vi "Mouse Up Event.vi"(4 "User Parameter":T1, 5 "Event Data":T3, 6 "PaneRef":refnum<vi>, 7 "Event Common Data":cluster{"Source":T4, "Type":T5, "Time":u32} {"Source" items=["LabVIEW UI"=0, "ActiveX"=1, "User Event"=25]}) -> ()   [LabVIEW 2020]
uses:
  <vilib>/event_ctls.llb/eventsource.ctl
  <vilib>/event_ctls.llb/lveventtype.ctl
  <vilib>/Utility/miscctls.llb/LVPoint32TypeDef.ctl
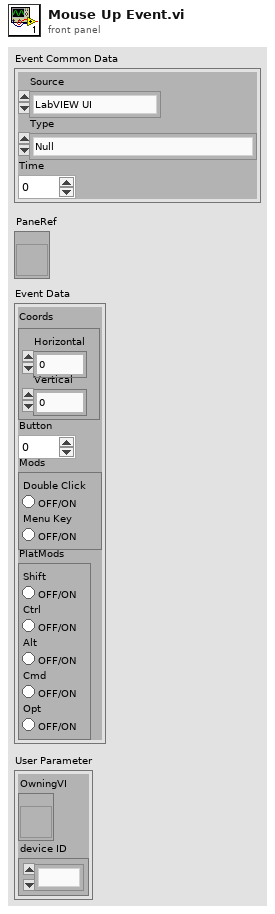
[diagram p1: front panel]
types:
  T1 = cluster{"OwningVI":refnum<vi>, "device ID":refnum<k1>}
  T2 = typedef "LVPoint32TypeDef.ctl" = cluster{"Horizontal":i32, "Vertical":i32}
  T3 = cluster{"Coords":T2, "Button":u16, "Mods":cluster{"Double Click":bool, "Menu Key":bool}, "PlatMods":cluster{"Shift":bool, "Ctrl":bool, "Alt":bool, "Cmd":bool, "Opt":bool}}
  T4 = typedef "eventsource.ctl" = u32
  T5 = typedef "lveventtype.ctl" = enum32{"Null", "Timeout", "Annotation Menu Selection", "Annotation Menu Selection?", "App Instance Close", "App Instance Close?", "Autoscale Range Change", "Bookmark Info Change", "Cell Edit", "Cell Edit?", "Cursor Grab", "Cursor Grab?", "Cursor Menu Selection", "Cursor Menu Selection?", "Cursor Move", "Cursor Release", "Data Change", "Direction Change", "Display State Change", "Drag Ended", "Drag Enter", "Drag Leave", "Drag Over", "Drag Source Update", "Drag Starting", "Drag Starting?", "Drop", "Exec State Change", "Key Down", "Key Down?", "Key Repeat", "Key Repeat?", "Key Up", "Listbox Double Click", "Menu Activation?", "Menu Selection (App)", "Menu Selection? (App)", "Menu Selection (User)", "Mouse Down", "Mouse Down?", "Mouse Enter", "Mouse Leave", "Mouse Move", "Mouse Up", "Mouse Wheel", "NI Security User Change (App)", "Pane Size", "Panel Close", "Panel Close?", "Panel Resize", "Plot Attribute Change", "Scale Range Change", "Shortcut Menu Activation?", "Shortcut Menu Selection (App)", "Shortcut Menu Selection? (App)", "Shortcut Menu Selection (User)", "Tree Double Click", "Tree Drag", "Tree Drag?", "Tree Drop", "Tree Drop?", "Tree Item Close", "Tree Item Close?", "Tree Item Open", "Tree Item Open?", "User Event", "Value Change"}
  T6 = typedef "LVRectTypeDef.ctl" = cluster{"Left":i16, "Top":i16, "Right":i16, "Bottom":i16}
  T7 = enum32{"Invalid", "Standard", "Closed", "Hidden", "Minimized", "Maximized"}
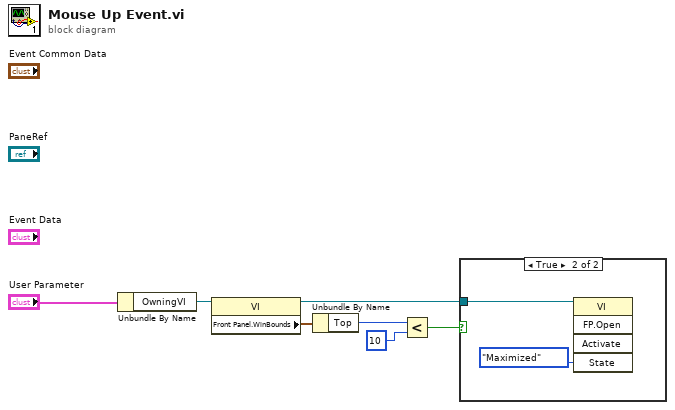
[diagram p0: block diagram]
diagram:
  n1 = Unbundle By Name("User Parameter") -> ("OwningVI"=w6:refnum<vi>)
  n2 = property class="VI"(reference=w6) -> (reference out=w2:refnum<vi>, "Front Panel.WinBounds"=w5:T6)  [unwired: 1 in, 1 out]
  n3 = Unbundle By Name(w5) -> ("Top"=w4:i16)
  n4 = Less?(x=w4, y=i16 10) -> (x < y?=w1:bool)
  n5 = case shown="True" w1 {
    tunnel: w2 -> [_ w9]
    frame False {
    }
    frame True {
      n6 = invoke class="VI" method="FP.Open"(reference=w9, "State"=T7."Maximized") -> ()  [unwired: 3 in, 5 out]
    }
  }
